vi "RW State Machine.vi"(8 "error in (no error)":errorcluster) -> (0 "error out":errorcluster)   [LabVIEW 2018]
uses:
  State Machine/State Machine.lvclass
  State Machine/State Machine.lvclass/State Machine.ctl
  <vilib>/addons/_JKI Toolkits/Caraya/classes/Assert/Assert.lvclass
  <vilib>/addons/_JKI Toolkits/Caraya/classes/Test/Test.lvclass
panel:
  in  "State Machine.lvclass":refnum<class "State Machine.lvclass">
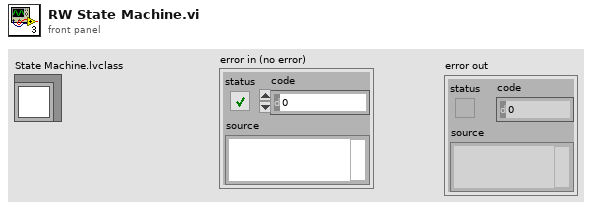
[diagram p1: front panel]
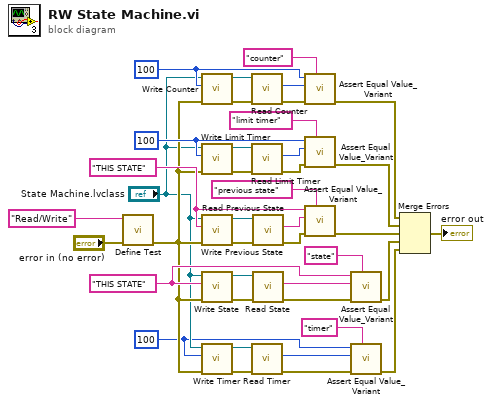
[diagram p0: block diagram]
diagram:
  w1 = 100
  w12 = "THIS STATE" ("Previous State")
  w20 = "THIS STATE" ("Previous State")
  w26 = 100
  w25 = 100
  n1 = call <vilib>:"Define Test.vi"("error in (no error)"="error in (no error)", "Label (VI Title)"="Read/Write") -> ("error out"=w5:errorcluster)  [unwired: 8 in, 1 out]
  n2 = call "Write Counter.vi"("error in (no error)"=w5, "Counter"=w26, "State Machine in"="State Machine.lvclass") -> ("error out"=w39:errorcluster, "State Machine out"=w40:refnum<class "State Machine.lvclass">)  [unwired: 7 in]
  n3 = call "Write Limit Timer.vi"("error in (no error)"=w5, "Limit Timer"=w25, "State Machine in"="State Machine.lvclass") -> ("error out"=w31:errorcluster, "State Machine out"=w27:refnum<class "State Machine.lvclass">)  [unwired: 7 in]
  n4 = call-dynamic "Write Previous State.vi"("error in (no error)"=w5, "Previous State"=w20, "State Machine in"="State Machine.lvclass") -> ("error out"=w23:errorcluster, "State Machine out"=w22:refnum<class "State Machine.lvclass">)  [unwired: 7 in]
  n5 = call-dynamic "Write State.vi"("error in (no error)"=w5, "State"=w12, "State Machine in"="State Machine.lvclass") -> ("error out"=w16:errorcluster, "State Machine out"=w15:refnum<class "State Machine.lvclass">)  [unwired: 7 in]
  n6 = call "Write Timer.vi"("error in (no error)"=w5, "Timer"=w1, "State Machine in"="State Machine.lvclass") -> ("error out"=w6:errorcluster, "State Machine out"=w3:refnum<class "State Machine.lvclass">)  [unwired: 7 in]
  n7 = call "Read Counter.vi"("error in (no error)"=w39, "State Machine in"=w40) -> ("error out"=w38:errorcluster, "Counter"=w37:u16)  [unwired: 7 in, 1 out]
  n8 = call "Read Limit Timer.vi"("error in (no error)"=w31, "State Machine in"=w27) -> ("error out"=w32:errorcluster, "Limit Timer"=w30:u32)  [unwired: 7 in, 1 out]
  n9 = call "Read Timer.vi"("error in (no error)"=w6, "State Machine in"=w3) -> ("error out"=w7:errorcluster, "Timer"=w2:u32)  [unwired: 7 in, 1 out]
  n10 = call-dynamic "Read Previous State.vi"("error in (no error)"=w23, "State Machine in"=w22) -> ("error out"=w24:errorcluster, "Previous State"=w21:string)  [unwired: 7 in, 1 out]
  n11 = call-dynamic "Read State.vi"("error in (no error)"=w16, "State Machine in"=w15) -> ("error out"=w14:errorcluster, "State"=w13:string)  [unwired: 7 in, 1 out]
  n12 = call <vilib>:"Assert Equal Value_Variant.vi"("Label"="counter", "error in (no error)"=w38, "Y"=w37, "X"=w26) -> ("error out"=w34:errorcluster)  [unwired: 6 in, 1 out]
  n13 = call <vilib>:"Assert Equal Value_Variant.vi"("Label"="limit timer", "error in (no error)"=w32, "Y"=w30, "X"=w25) -> ("error out"=w33:errorcluster)  [unwired: 6 in, 1 out]
  n14 = call <vilib>:"Assert Equal Value_Variant.vi"("Label"="previous state", "error in (no error)"=w24, "Y"=w21, "X"=w20) -> ("error out"=w18:errorcluster)  [unwired: 6 in, 1 out]
  n15 = call <vilib>:"Assert Equal Value_Variant.vi"("Label"="state", "error in (no error)"=w14, "Y"=w13, "X"=w12) -> ("error out"=w17:errorcluster)  [unwired: 6 in, 1 out]
  n16 = call <vilib>:"Assert Equal Value_Variant.vi"("Label"="timer", "error in (no error)"=w7, "Y"=w2, "X"=w1) -> ("error out"=w9:errorcluster)  [unwired: 6 in, 1 out]
  n17 = Merge Errors(w34, w33, w18, w17, w9) -> (→"error out":errorcluster)
